vi "HandleTCP.vi"(8 "error in (no error)":errorcluster, 11 "connection ID":refnum<k5>) -> ()   [LabVIEW 2014]
panel:
  out "error out":errorcluster
  out "number":i32
  out "data out":string
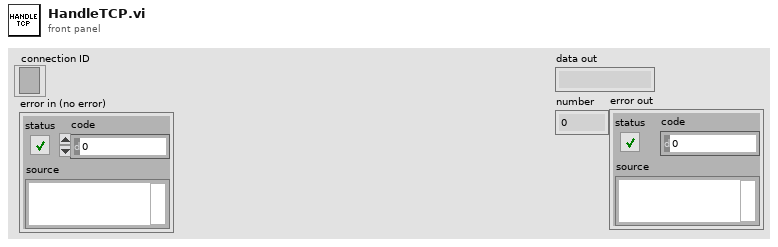
[diagram p1: front panel]
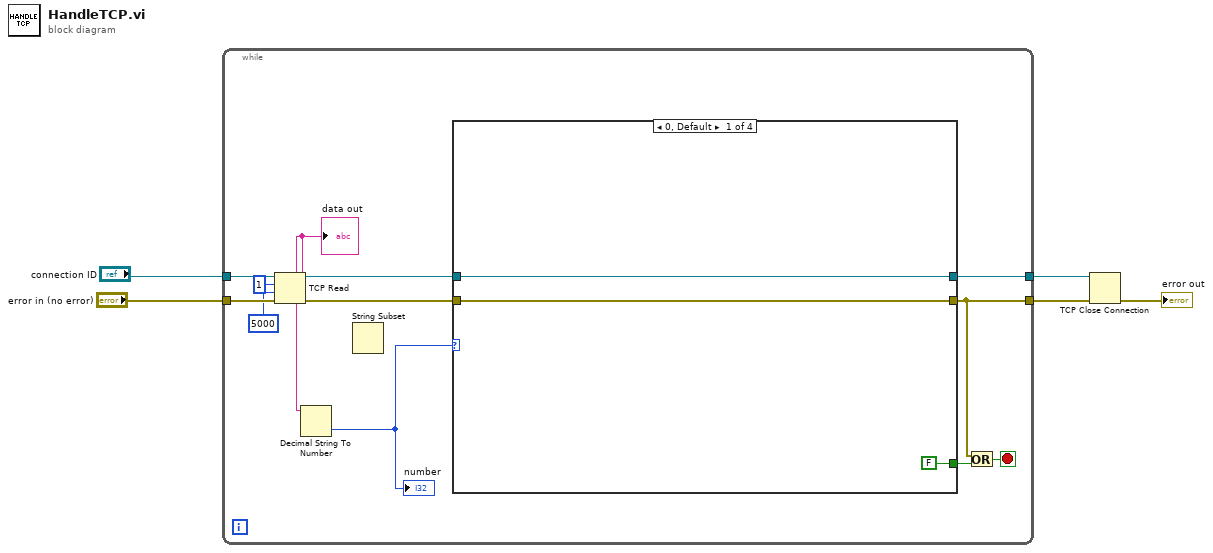
[diagram p0: block diagram]
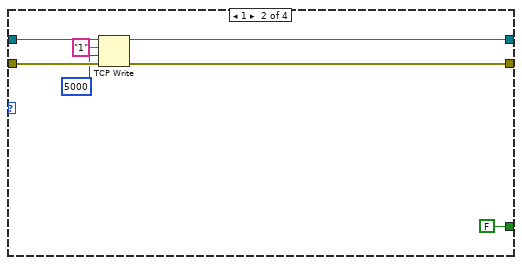
[diagram p2: hidden frame]
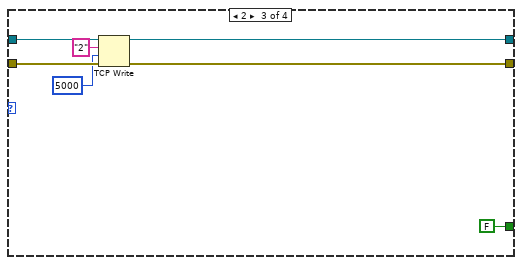
[diagram p3: hidden frame]
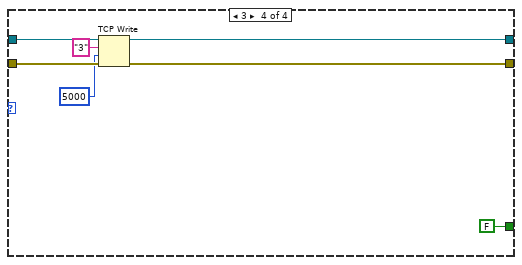
[diagram p4: hidden frame]
diagram:
  n1 = while {
    tunnel: "connection ID" -> [w16]
    tunnel: "error in (no error)" -> [w15]
    tunnel: [w8] -> w2
    tunnel: [w11] -> w3
    stop <- w9 stop-if-true
    n2 = TCP Read(connection ID=w16, bytes to read=1, error in (no error)=w15, 9:5000 ("timeout ms (25000)")) -> (connection ID out=w13:refnum<k5>, data out=w7:string, error out=w14:errorcluster)  [unwired: 1 in]
    "data out" <- w7
    n3 = Decimal String To Number(string=w7) -> (number=w6:i32)  [unwired: 2 in, 1 out]
    "number" <- w6
    n4 = String Subset() -> ()  [unwired: 3 in, 1 out]
    n5 = case shown="0, Default" w6 {
      tunnel: w14 -> [w19 w27 w34 w41]
      tunnel: w13 -> [w20 w26 w33 w40]
      tunnel: [w20 w24 w31 w38] -> w11
      tunnel: [w19 w25 w32 w39] -> w8
      tunnel: [FALSE FALSE FALSE FALSE] -> w12
      frame 0, Default {
      }
      frame 1 {
        n6 = TCP Write(connection ID=w26, data in="1", error in (no error)=w27, 9:5000 ("timeout ms (25000)")) -> (connection ID out=w24:refnum<k5>, error out=w25:errorcluster)  [unwired: 1 out]
      }
      frame 2 {
        n7 = TCP Write(connection ID=w33, data in="2", error in (no error)=w34, 9:5000 ("timeout ms (25000)")) -> (connection ID out=w31:refnum<k5>, error out=w32:errorcluster)  [unwired: 1 out]
      }
      frame 3 {
        n8 = TCP Write(connection ID=w40, data in="3", error in (no error)=w41, 9:5000 ("timeout ms (25000)")) -> (connection ID out=w38:refnum<k5>, error out=w39:errorcluster)  [unwired: 1 out]
      }
    }
    n9 = Or(x=w8, y=w12) -> (x .or. y?=w9:bool)
  }
  n10 = TCP Close Connection(connection ID=w3, error in (no error)=w2) -> (error out=→"error out":errorcluster)  [unwired: 1 in, 1 out]
